vi "设置窗口.vi"() -> (2 "连接配置":T1={"连接类型"=enum."串口", "串口"="", "IP"="192.168.1.205", "PORT"="502"}, 3 "确定输出":bool)   [LabVIEW 2016, in "重金属.lvlib"]
panel:
  in  "连接类型":enum16{"串口", "TCP"}(ring)
  out "选板":enum32{"串口", "TCP"}(tab)
  in  "串口":refnum<visa-resource-name>
  in  "IP":string="192.168.1.205"
  in  "PORT":string="502"
  in  "取消":bool
  in  "确定":bool
  # "请选择相应的串口号"
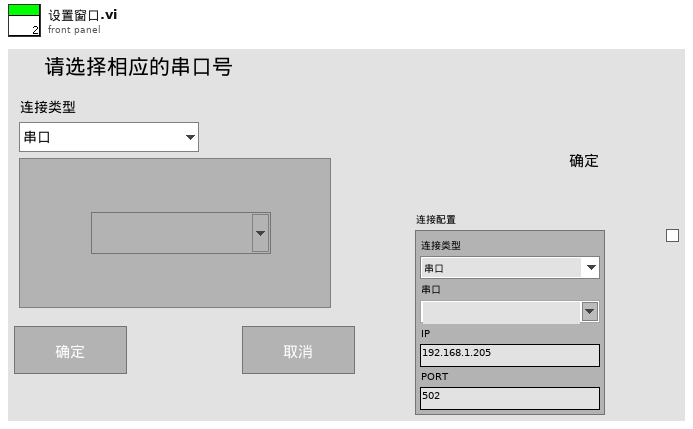
[diagram p1: front panel]
types:
  T1 = cluster{"连接类型":enum16{"串口", "TCP"}, "串口":string, "IP":string, "PORT":string}
  T2 = cluster{"连接类型":enum16{"串口", "TCP"}, "串口":refnum<visa-resource-name>, "IP":string, "PORT":string}
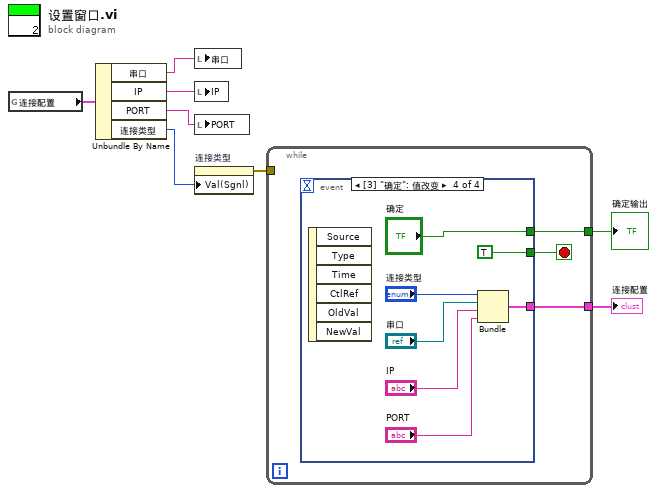
[diagram p0: block diagram]
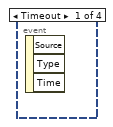
[diagram p2: hidden frame]
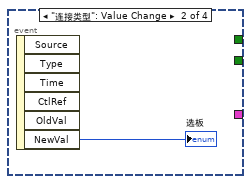
[diagram p3: hidden frame]
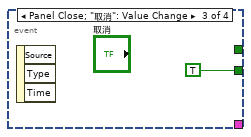
[diagram p4: hidden frame]
diagram:
  n1 = global read "全局变量.vi" "连接配置"() -> (w6:T1)
  n2 = Unbundle By Name(w6) -> ("串口"=w5:string, "IP"=w3:string, "PORT"=w2:string, "连接类型"=w4:enum16{"串口", "TCP"})
  n3 = local write "串口"(w5) -> ()
  n4 = local write "IP"(w3) -> ()
  n5 = local write "PORT"(w2) -> ()
  n6 = property on="连接类型" class="Enum (严格)"("Val(Sgnl)"=w4) -> (error out=w1:errorcluster)  [unwired: 2 in, 1 out]
  n7 = while {
    tunnel: [w10] -> w8
    tunnel: [w9] -> w7
    tunnel: w1 -> [_]
    stop <- w11 stop-if-true
    n8 = event shown="[3] \"确定\": 值改变" {
      selector: _ -> [_ _ _ _]
      dyn-events: _ -> [_ _ _ _]
      timeout: _ -> [_ _ _ _]
      tunnel: [_ _ TRUE TRUE] -> w11
      tunnel: [_ _ _ "确定"] -> w10
      tunnel: [_ _ _ w14] -> w9
      event Timeout {
        n9 = event-data() -> ()  [unwired: 1 in, 3 out]
      }
      event "连接类型": Value Change {
        n10 = event-data() -> ("NewVal"=→"选板":enum16{"串口", "TCP"})  [unwired: 1 in, 5 out]
      }
      event Panel Close; "取消": Value Change {
        n11 = event-data() -> ()  [unwired: 1 in, 3 out]
      }
      event "确定": Value Change {
        n12 = event-data() -> ()  [unwired: 1 in, 6 out]
        n13 = Bundle("连接类型"="连接类型", "串口"="串口", "IP"="IP", "PORT"="PORT") -> (w14:T2)  [unwired: 1 in]
      }
    }
  }
  "确定输出" <- w8
  "连接配置" <- w7
